vi "Keithley Report2400.vi"(0 "Test operator":string="Operator's name", 1 "Start":string="100", 2 "AppArray":bool[](array[boolean])=[FALSE, FALSE, FALSE, FALSE, FALSE, FALSE, FALSE, FALSE, FALSE, FALSE, FALSE, FALSE, FALSE, FALSE, FALSE, FALSE, FALSE, FALSE, FALSE, FALSE], 3 "Cluster":T1={"A 3"=[["100", "41.7", "38.5"], ["125", "41.7", "35.2"], ["160", "41.5", "37.5"], ["200", "42.3", "42.5"], ["250", "46.9", "46.8"], ["315", "51.9", "52.6"], ["400", "52.3", "46.7"], ["500  ", "46.5", "41.6"], ["630", "42.3", "35.9"], ["800", "41.1", "32.6"]], "A 4"=[["100", "41.7", "38.5"], ["125", "41.7", "35.2"], ["160", "41.5", "37.5"], ["200", "42.3", "42.5"], ["250", "46.9", "46.8"], ["315", "51.9", "52.6"], ["400", "52.3", "46.7"], ["500  ", "46.5", "41.6"], ["630", "42.3", "35.9"], ["800", "41.1", "32.6"]], "A 5"=[["100", "41.7", "38.5"], ["125", "41.7", "35.2"], ["160", "41.5", "37.5"], ["200", "42.3", "42.5"], ["250", "46.9", "46.8"], ["315", "51.9", "52.6"], ["400", "52.3", "46.7"], ["500  ", "46.5", "41.6"], ["630", "42.3", "35.9"], ["800", "41.1", "32.6"]], "A 6"=[["100", "41.7", "38.5"], ["125", "41.7", "35.2"], ["160", "41.5", "37.5"], ["200", "42.3", "42.5"], ["250", "46.9", "46.8"], ["315", "51.9", "52.6"], ["400", "52.3", "46.7"], ["500  ", "46.5", "41.6"], ["630", "42.3", "35.9"], ["800", "41.1", "32.6"]], "A 7"=[["100", "41.7", "38.5"], ["125", "41.7", "35.2"], ["160", "41.5", "37.5"], ["200", "42.3", "42.5"], ["250", "46.9", "46.8"], ["315", "51.9", "52.6"], ["400", "52.3", "46.7"], ["500  ", "46.5", "41.6"], ["630", "42.3", "35.9"], ["800", "41.1", "32.6"]], "A 8"=[["100", "41.7", "38.5"], ["125", "41.7", "35.2"], ["160", "41.5", "37.5"], ["200", "42.3", "42.5"], ["250", "46.9", "46.8"], ["315", "51.9", "52.6"], ["400", "52.3", "46.7"], ["500  ", "46.5", "41.6"], ["630", "42.3", "35.9"], ["800", "41.1", "32.6"]], "A 9"=[["100", "41.7", "38.5"], ["125", "41.7", "35.2"], ["160", "41.5", "37.5"], ["200", "42.3", "42.5"], ["250", "46.9", "46.8"], ["315", "51.9", "52.6"], ["400", "52.3", "46.7"], ["500  ", "46.5", "41.6"], ["630", "42.3", "35.9"], ["800", "41.1", "32.6"]], "A 10"=[["100", "41.7", "38.5"], ["125", "41.7", "35.2"], ["160", "41.5", "37.5"], ["200", "42.3", "42.5"], ["250", "46.9", "46.8"], ["315", "51.9", "52.6"], ["400", "52.3", "46.7"], ["500  ", "46.5", "41.6"], ["630", "42.3", "35.9"], ["800", "41.1", "32.6"]], "A 11"=[["100", "41.7", "38.5"], ["125", "41.7", "35.2"], ["160", "41.5", "37.5"], ["200", "42.3", "42.5"], ["250", "46.9", "46.8"], ["315", "51.9", "52.6"], ["400", "52.3", "46.7"], ["500  ", "46.5", "41.6"], ["630", "42.3", "35.9"], ["800", "41.1", "32.6"]], "A 12"=[["100", "41.7", "38.5"], ["125", "41.7", "35.2"], ["160", "41.5", "37.5"], ["200", "42.3", "42.5"], ["250", "46.9", "46.8"], ["315", "51.9", "52.6"], ["400", "52.3", "46.7"], ["500  ", "46.5", "41.6"], ["630", "42.3", "35.9"], ["800", "41.1", "32.6"]], "A 13"=[["100", "41.7", "38.5"], ["125", "41.7", "35.2"], ["160", "41.5", "37.5"], ["200", "42.3", "42.5"], ["250", "46.9", "46.8"], ["315", "51.9", "52.6"], ["400", "52.3", "46.7"], ["500  ", "46.5", "41.6"], ["630", "42.3", "35.9"], ["800", "41.1", "32.6"]], "A 14"=[["100", "41.7", "38.5"], ["125", "41.7", "35.2"], ["160", "41.5", "37.5"], ["200", "42.3", "42.5"], ["250", "46.9", "46.8"], ["315", "51.9", "52.6"], ["400", "52.3", "46.7"], ["500  ", "46.5", "41.6"], ["630", "42.3", "35.9"], ["800", "41.1", "32.6"]], "A 15"=[["100", "41.7", "38.5"], ["125", "41.7", "35.2"], ["160", "41.5", "37.5"], ["200", "42.3", "42.5"], ["250", "46.9", "46.8"], ["315", "51.9", "52.6"], ["400", "52.3", "46.7"], ["500  ", "46.5", "41.6"], ["630", "42.3", "35.9"], ["800", "41.1", "32.6"]], "A 16"=[["100", "41.7", "38.5"], ["125", "41.7", "35.2"], ["160", "41.5", "37.5"], ["200", "42.3", "42.5"], ["250", "46.9", "46.8"], ["315", "51.9", "52.6"], ["400", "52.3", "46.7"], ["500  ", "46.5", "41.6"], ["630", "42.3", "35.9"], ["800", "41.1", "32.6"]], "A 17"=[["100", "41.7", "38.5"], ["125", "41.7", "35.2"], ["160", "41.5", "37.5"], ["200", "42.3", "42.5"], ["250", "46.9", "46.8"], ["315", "51.9", "52.6"], ["400", "52.3", "46.7"], ["500  ", "46.5", "41.6"], ["630", "42.3", "35.9"], ["800", "41.1", "32.6"]], "A 18"=[["100", "41.7", "38.5"], ["125", "41.7", "35.2"], ["160", "41.5", "37.5"], ["200", "42.3", "42.5"], ["250", "46.9", "46.8"], ["315", "51.9", "52.6"], ["400", "52.3", "46.7"], ["500  ", "46.5", "41.6"], ["630", "42.3", "35.9"], ["800", "41.1", "32.6"]], "A 19"=[["100", "41.7", "38.5"], ["125", "41.7", "35.2"], ["160", "41.5", "37.5"], ["200", "42.3", "42.5"], ["250", "46.9", "46.8"], ["315", "51.9", "52.6"], ["400", "52.3", "46.7"], ["500  ", "46.5", "41.6"], ["630", "42.3", "35.9"], ["800", "41.1", "32.6"]], "A 20"=[["100", "41.7", "38.5"], ["125", "41.7", "35.2"], ["160", "41.5", "37.5"], ["200", "42.3", "42.5"], ["250", "46.9", "46.8"], ["315", "51.9", "52.6"], ["400", "52.3", "46.7"], ["500  ", "46.5", "41.6"], ["630", "42.3", "35.9"], ["800", "41.1", "32.6"]], "A 1"=[["100", "41.7", "38.5"], ["125", "41.7", "35.2"], ["160", "41.5", "37.5"], ["200", "42.3", "42.5"], ["250", "46.9", "46.8"], ["315", "51.9", "52.6"], ["400", "52.3", "46.7"], ["500  ", "46.5", "41.6"], ["630", "42.3", "35.9"], ["800", "41.1", "32.6"]], "A 2"=[["100", "41.7", "38.5"], ["125", "41.7", "35.2"], ["160", "41.5", "37.5"], ["200", "42.3", "42.5"], ["250", "46.9", "46.8"], ["315", "51.9", "52.6"], ["400", "52.3", "46.7"], ["500  ", "46.5", "41.6"], ["630", "42.3", "35.9"], ["800", "41.1", "32.6"]]}, 4 "Stop":string="Operator's name", 5 "Step":string="20", 7 "Compliance":string="70", 8 "Data":string[][](table)=[["100", "41.7", "38.5"], ["125", "41.7", "35.2"], ["160", "41.5", "37.5"], ["200", "42.3", "42.5"], ["250", "46.9", "46.8"], ["315", "51.9", "52.6"], ["400", "52.3", "46.7"], ["500  ", "46.5", "41.6"], ["630", "42.3", "35.9"], ["800", "41.1", "32.6"]], 10 "Comp Unit":string="Operator's name", 11 "DataPoints":string="Operator's name", 12 "Ctl Refnum":refnum<vi>, 13 "Start unit":string="100", 14 "test time":timestamp, 18 "Stop Unit":string="Operator's name", 19 "StepUnit":string="20") -> ()   [LabVIEW 2017]
doc: "This example shows how to generate a report from a template. The template contains a preformatted table and a preformatted graph which are updated with Append Table to Report.vi and Excel Update Graph.vi."
uses:
  <vilib>/addons/_office/_exclsub.llb/font.ctl
  <vilib>/Utility/NIReport.llb/image depth.ctl
  TCH Golbal.vi
  <vilib>/Utility/NIReport.llb/Append Report Text (str wrap).vi
  <vilib>/Utility/NIReport.llb/Append Text Table to Report (wrap).vi
  <vilib>/Utility/NIReport.llb/NI_report.lvclass
  <vilib>/Utility/NIReport.llb/NI_ReportGenerationCore.lvlib
  <vilib>/Utility/NIReport.llb/Excel/NI_Excel.lvclass
  <vilib>/addons/_office/NI_ReportGenerationToolkit.lvlib
panel:
  in  "Express VI?":bool
  # "Overview: This example shows how to generate a report from a template using either the Excel Report Generation VIs or the MS Office Report Express VI.\nRequirements: Report Generation Toolkit, Microsoft Excel\nInstructions:\nRun the VI."
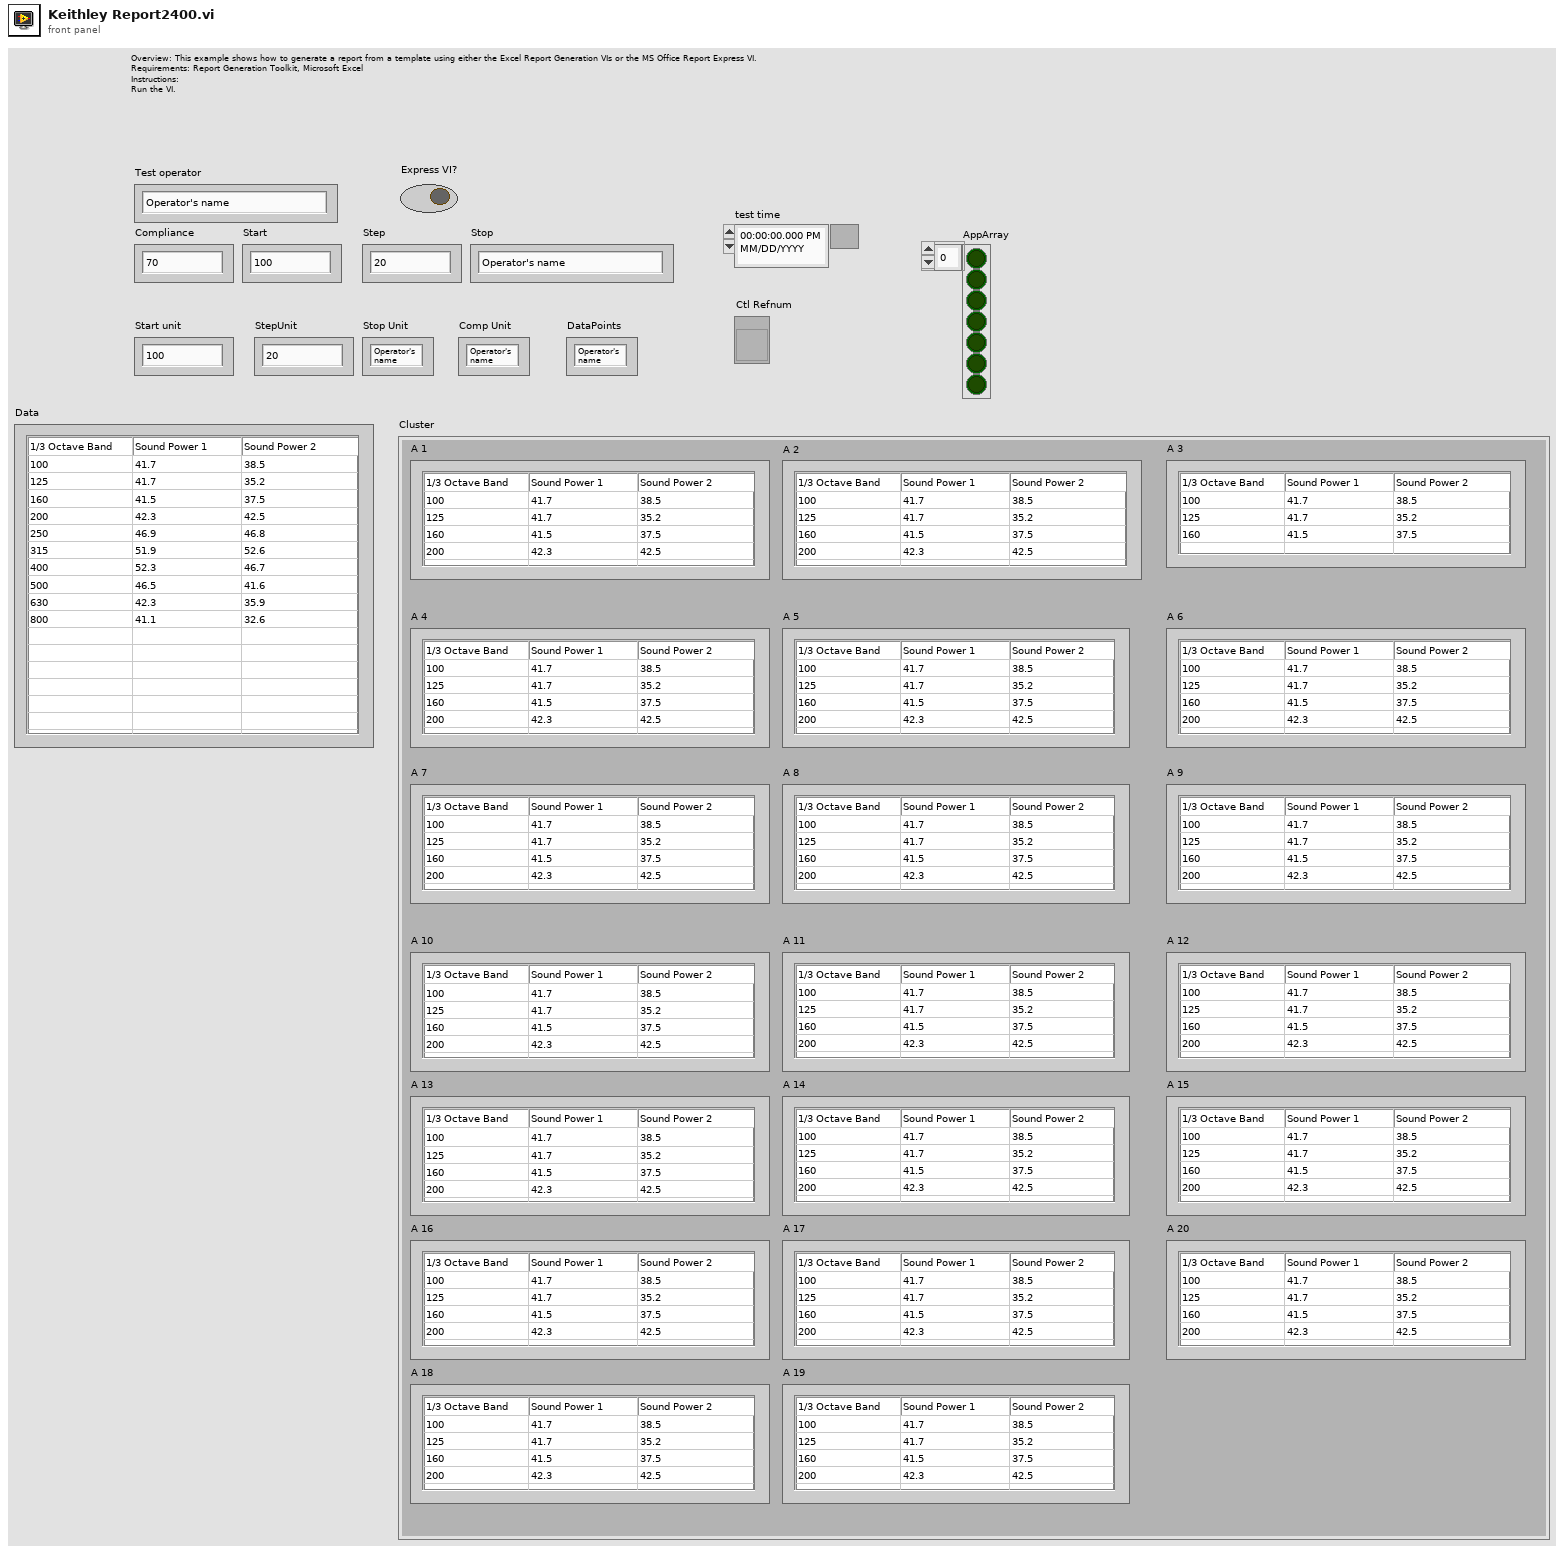
[diagram p1: front panel]
types:
  T1 = cluster{"A 3":string[][], "A 4":string[][], "A 5":string[][], "A 6":string[][], "A 7":string[][], "A 8":string[][], "A 9":string[][], "A 10":string[][], "A 11":string[][], "A 12":string[][], "A 13":string[][], "A 14":string[][], "A 15":string[][], "A 16":string[][], "A 17":string[][], "A 18":string[][], "A 19":string[][], "A 20":string[][], "A 1":string[][], "A 2":string[][]}
  T2 = cluster{"position (Excel)":cluster{"row":i32, "column":i32}, "name (Excel)":string, "bookmark (Word)":string}
  T3 = cluster{"position (excel)":cluster{"row":i32, "column":i32}, "name (excel)":string, "bookmark (word)":string}
  T4 = cluster{"position (Excel)":cluster{"row":i32, "column":i32}, "name (Excel)":string, string}
  T5 = enum16{"Standard Report", "HTML", "Word", "Excel"}
  T6 = enum32{"invalid app kind", "Development System", "Run Time System", "Student Edition", "Embedded LabVIEW", "Evaluation", "Custom"}
  T7 = typedef "NI_ReportGenerationToolkit.lvlib/font.ctl" = cluster{"font name":string, "font size":dbl, "bold":u16, "italic":u16, "underline":u16, "strike through":u16, "font color":u32}
  T8 = cluster{"start (wd) - row (xl) ":i32, "end (wd) - col (xl) ":i32}
  T9 = typedef "NI_ReportGenerationCore.lvlib/image depth.ctl" = u16
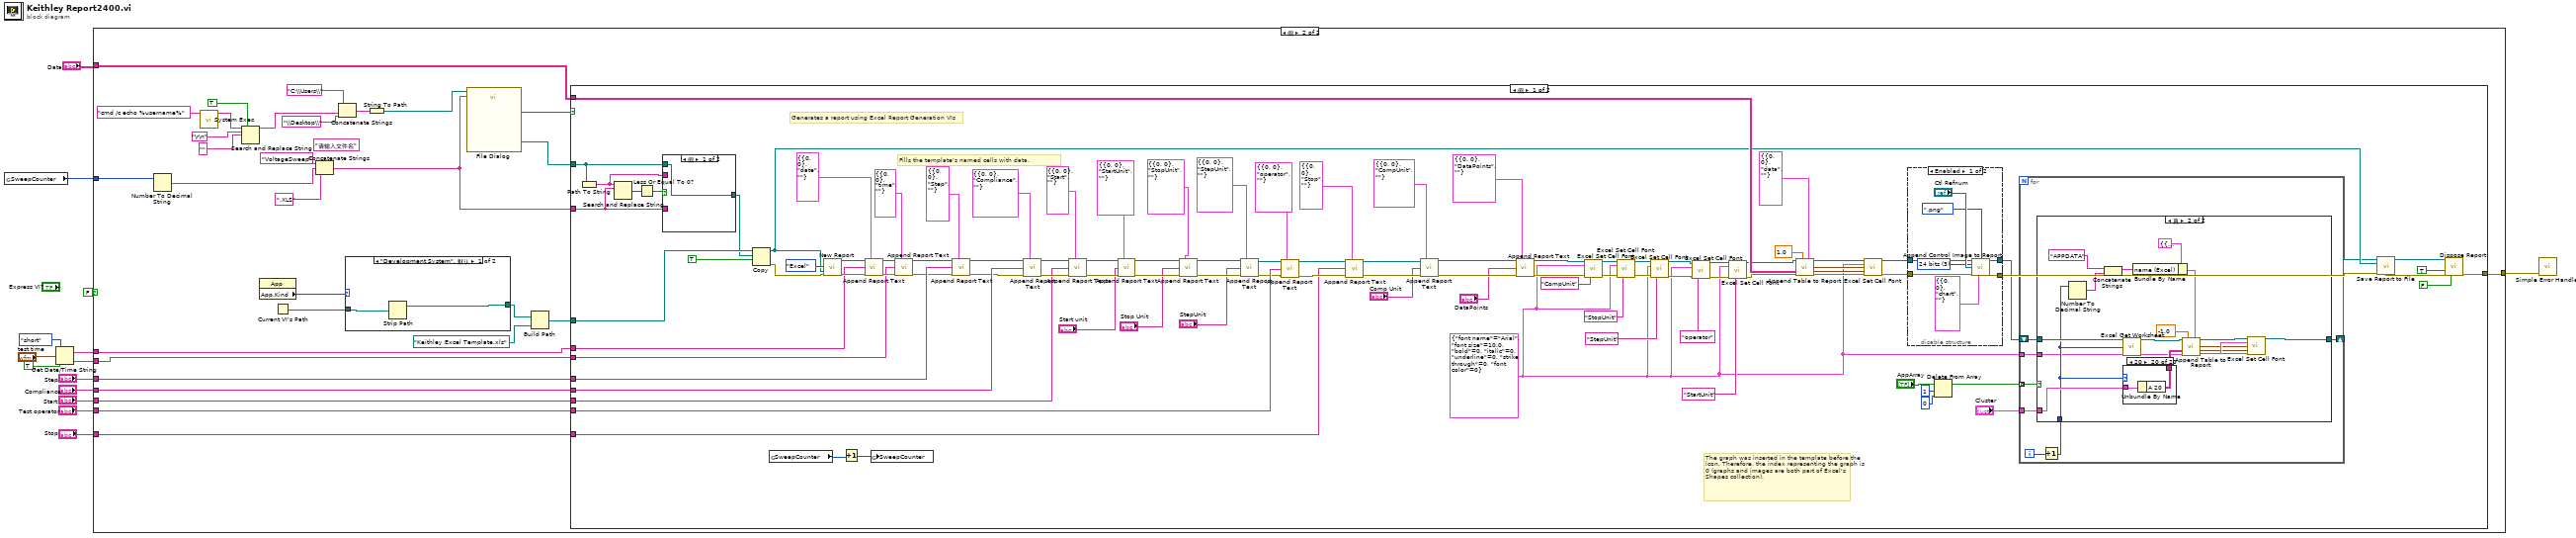
[diagram p0: block diagram]
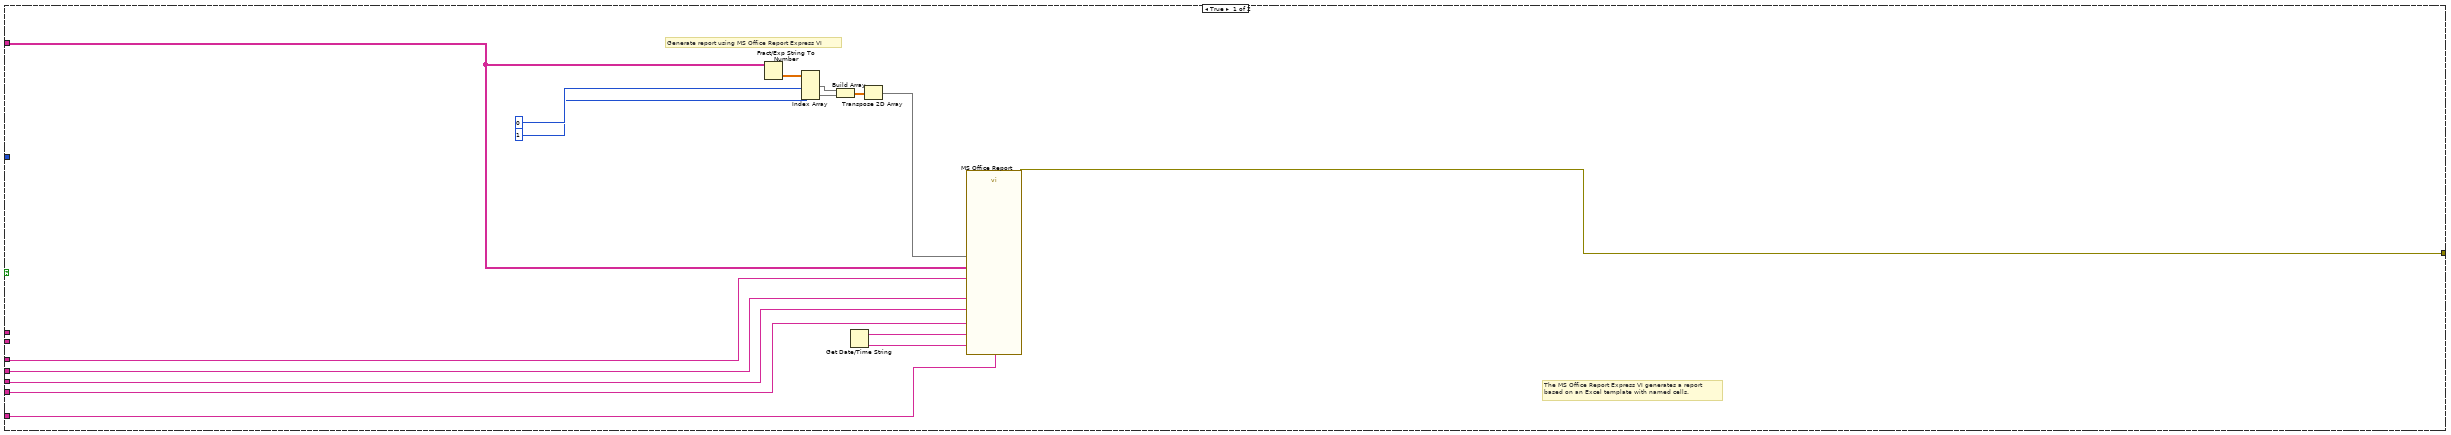
[diagram p2: hidden frame]
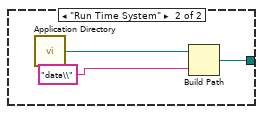
[diagram p3: hidden frame]
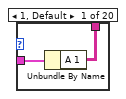
[diagram p6: hidden frame]
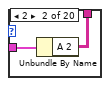
[diagram p7: hidden frame]
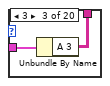
[diagram p8: hidden frame]
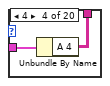
[diagram p9: hidden frame]
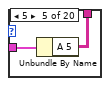
[diagram p10: hidden frame]
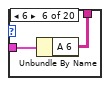
[diagram p11: hidden frame]
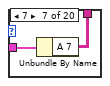
[diagram p12: hidden frame]
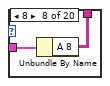
[diagram p13: hidden frame]
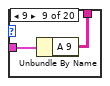
[diagram p14: hidden frame]
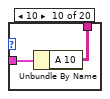
[diagram p15: hidden frame]
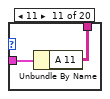
[diagram p16: hidden frame]
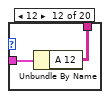
[diagram p17: hidden frame]
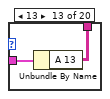
[diagram p18: hidden frame]
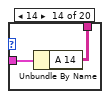
[diagram p19: hidden frame]
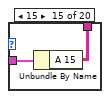
[diagram p20: hidden frame]
diagram:
  n1 = global read "TCH Golbal.vi" "SweepCounter"() -> (w1:i32)
  n2 = Get Date/Time String(date format (0)=enum16{"short", "long", "abbreviated"}."short", seconds (now)="test time", want seconds? (F)=TRUE) -> (date string=w5:string, time string=w4:string)
  n3 = case shown="假" FALSE ("Express VI?") {
    tunnel: "Step" -> [w29 w61]
    tunnel: "Compliance" -> [w23 w60]
    tunnel: "Start" -> [w28 w56]
    tunnel: "Test operator" -> [w27 w55]
    tunnel: [w30 w59] -> w10
    tunnel: "Data" -> [w26 w58]
    tunnel: "Stop" -> [w22 w31]
    tunnel: w5 -> [_ w53]
    tunnel: w4 -> [_ w32]
    tunnel: w1 -> [_ w51]
    frame True {
      # "Generate report using MS Office Report Express VI"
      # "The MS Office Report Express VI generates a report\nbased on an Excel template with named cells."
      n4 = Fract/Exp String To Number(string=w26) -> (number=w21:dbl[][])  [unwired: 3 in, 1 out]
      n5 = Index Array(array=w21, index (col) #1=0 ("disabled index (col)"), index (col) #2=1 ("index (col)")) -> (element #1=w18:dbl[], element #2=w17:dbl[])  [unwired: 2 in]
      n6 = Build Array(w18, w17) -> (w16:dbl[][])
      n7 = Get Date/Time String() -> (date string=w24:string, time string=w25:string)  [unwired: 3 in]
      n8 = Transpose 2D Array(2D array=w16) -> (transposed array=w15:dbl[][])
      n9 = call "MS Office Report"("chart"=w15, "Compliance"=w23, "data"=w26, "date"=w24, "operator"=w27, "Start"=w28, "Step"=w29, "Stop"=w22, "time"=w25) -> ("error out"=w30:errorcluster)  [unwired: 18 in]
    }
    frame False {
      (unwired) "请输入文件名" ("prompt")
      n10 = Number To Decimal String(number=w51) -> (decimal integer string=w50:string)  [unwired: 1 in]
      n11 = call <vilib>:"System Exec.vi"("command line"="cmd /c echo %username%") -> ("standard output"=w42:string)  [unwired: 7 in, 3 out]
      n12 = Search and Replace String(replace all?=TRUE ("replace all? (F)"), input string=w42, search string="\r\n", replace string="" ("replace string (\"\")")) -> (result string=w41:string)  [unwired: 4 in, 3 out]
      n13 = property class="App"() -> ("App.Kind"=w49:T6)  [unwired: 2 in, 2 out]
      n14 = Current VI's Path() -> (path=w34:path)
      n15 = Concatenate Strings("VoltageSweep" ("filename"), w50, ".XLS" ("default name")) -> (w35:string)
      n16 = Concatenate Strings("C:\\Users\\" ("string"), w41, "\\Desktop\\" ("string")) -> (w46:string)
      n17 = case shown="\"Development System\", 默认" w49 {
        tunnel: [w62 w65] -> w33
        tunnel: w34 -> [w63 _]
        frame "Development System", Default {
          n18 = Strip Path(path=w63) -> (stripped path=w62:path)  [unwired: 1 out]
        }
        frame "Run Time System" {
          n19 = call <vilib>:"Application Directory.vi"() -> ("Application Directory"=w64:path)
          n20 = Build Path(base path=w64, name or relative path="data\\") -> (appended path=w65:path)
        }
      }
      n21 = String To Path(string=w46) -> (path=w37:path)
      n22 = call "File Dialog"("start path"=w37, "default name"=w35) -> ("selected path"=w39:path, "cancelled"=w36:bool)  [unwired: 10 in, 2 out]
      n23 = Build Path(base path=w33, name or relative path=path "Keithley Excel Template.xls") -> (appended path=w54:path)
      n24 = case shown="假" w36 {
        tunnel: w61 -> [w167 _]
        tunnel: w60 -> [w166 _]
        tunnel: [w106 _] -> w59
        tunnel: w58 -> [w149 _]
        tunnel: w31 -> [w146 _]
        tunnel: w56 -> [w144 _]
        tunnel: w55 -> [w141 _]
        tunnel: w54 -> [w112 _]
        tunnel: w53 -> [w111 _]
        tunnel: w32 -> [w110 _]
        tunnel: w39 -> [w99 _]
        tunnel: w35 -> [w100 _]
        frame False {
          w67 = T7 {"font name"="Arial", "font size"=10.0, "bold"=0, "italic"=0, "underline"=0, "strike through"=0, "font color"=0} ("font")
          # "Fills the template's named cells with data."
          # "The graph was inserted in the template before the icon. Therefore, the index representing the graph is 0 (graphs and images are both part of Excel's Shapes collection)."
          # "Generates a report using Excel Report Generation VIs"
          n25 = Path To String(path=w99) -> (string=w74:string)
          n26 = Search and Replace String(input string=w74, search string=w100) -> (number of replacements=w97:i32)  [unwired: 6 in, 3 out]
          n27 = Less Or Equal To 0?(x=w97) -> (x <= 0?=w101:bool)
          n28 = case shown="假" w101 {
            tunnel: w99 -> [w242 _]
            tunnel: w100 -> [_ _]
            tunnel: [w242 w243] -> w98
            tunnel: w74 -> [_ w246]
            frame False {
            }
            frame True {
              n29 = Concatenate Strings(w246, ".xls" ("string")) -> (w244:string)
              n30 = String To Path(string=w244) -> (path=w243:path)
            }
          }
          n31 = Copy(9:TRUE ("overwrite (F)"), 10:w98, 11:w112) -> (0:w102:errorcluster, 3:w103:path)  [unwired: 2 in, 1 out]
          n32 = global read "TCH Golbal.vi" "SweepCounter"() -> (w109:i32)
          n33 = call <vilib>:"New Report.vi"("report type"=T5."Excel", "template (empty)"=w103, "error in (no error)"=w102) -> ("report out"=w159:refnum<class "NI_report.lvclass">, "error out"=w164:errorcluster)  [unwired: 11 in]
          n34 = Increment(x=w109) -> (x+1=w108:i32)
          n35 = call-poly <vilib>:"Append Report Text.vi"("report in"=w159, "MS Office parameters"=T2 {"position (Excel)"={"row"=0, "column"=0}, "name (Excel)"="date", "bookmark (Word)"=""}, "text"=w111, "error in (no error)"=w164) -> ("report out"=w158:refnum<class "NI_report.lvclass">, "error out"=w163:errorcluster)  [unwired: 8 in, 2 out]
          n36 = global write "TCH Golbal.vi" "SweepCounter"(w108) -> ()
          n37 = call-poly <vilib>:"Append Report Text.vi"("report in"=w158, "MS Office parameters"=T2 {"position (Excel)"={"row"=0, "column"=0}, "name (Excel)"="time", "bookmark (Word)"=""}, "text"=w110, "error in (no error)"=w163) -> ("report out"=w157:refnum<class "NI_report.lvclass">, "error out"=w162:errorcluster)  [unwired: 8 in, 2 out]
          n38 = call-poly <vilib>:"Append Report Text.vi"("report in"=w157, "MS Office parameters"=T3 {"position (excel)"={"row"=0, "column"=0}, "name (excel)"="Step", "bookmark (word)"=""}, "text"=w167, "error in (no error)"=w162) -> ("report out"=w156:refnum<class "NI_report.lvclass">, "error out"=w161:errorcluster)  [unwired: 8 in, 2 out]
          n39 = call-poly <vilib>:"Append Report Text.vi"("report in"=w156, "MS Office parameters"=T2 {"position (Excel)"={"row"=0, "column"=0}, "name (Excel)"="Compliance", "bookmark (Word)"=""}, "text"=w166, "error in (no error)"=w161) -> ("report out"=w155:refnum<class "NI_report.lvclass">, "error out"=w160:errorcluster)  [unwired: 8 in, 2 out]
          n40 = call-poly <vilib>:"Append Report Text.vi"("report in"=w155, "MS Office parameters"=T2 {"position (Excel)"={"row"=0, "column"=0}, "name (Excel)"="Start", "bookmark (Word)"=""}, "text"=w144, "error in (no error)"=w160) -> ("report out"=w140:refnum<class "NI_report.lvclass">, "error out"=w139:errorcluster)  [unwired: 8 in, 2 out]
          n41 = call-poly <vilib>:"Append Report Text.vi"("report in"=w140, "MS Office parameters"=T3 {"position (excel)"={"row"=0, "column"=0}, "name (excel)"="StartUnit", "bookmark (word)"=""}, "text"="Start unit", "error in (no error)"=w139) -> ("report out"=w138:refnum<class "NI_report.lvclass">, "error out"=w137:errorcluster)  [unwired: 8 in, 2 out]
          n42 = call-poly <vilib>:"Append Report Text.vi"("report in"=w138, "MS Office parameters"=T3 {"position (excel)"={"row"=0, "column"=0}, "name (excel)"="StopUnit", "bookmark (word)"=""}, "text"="Stop Unit", "error in (no error)"=w137) -> ("report out"=w136:refnum<class "NI_report.lvclass">, "error out"=w135:errorcluster)  [unwired: 8 in, 2 out]
          n43 = call-poly <vilib>:"Append Report Text.vi"("report in"=w136, "MS Office parameters"=T3 {"position (excel)"={"row"=0, "column"=0}, "name (excel)"="StepUnit", "bookmark (word)"=""}, "text"="StepUnit", "error in (no error)"=w135) -> ("report out"=w114:refnum<class "NI_report.lvclass">, "error out"=w116:errorcluster)  [unwired: 8 in, 2 out]
          n44 = call-poly <vilib>:"Append Report Text.vi"("report in"=w114, "MS Office parameters"=T2 {"position (Excel)"={"row"=0, "column"=0}, "name (Excel)"="operator", "bookmark (Word)"=""}, "text"=w141, "error in (no error)"=w116) -> ("report out"=w148:refnum<class "NI_report.lvclass">, "error out"=w147:errorcluster)  [unwired: 8 in, 2 out]
          n45 = call-poly <vilib>:"Append Report Text.vi"("report in"=w148, "MS Office parameters"=T2 {"position (Excel)"={"row"=0, "column"=0}, "name (Excel)"="Stop", "bookmark (Word)"=""}, "text"=w146, "error in (no error)"=w147) -> ("report out"=w92:refnum<class "NI_report.lvclass">, "error out"=w91:errorcluster)  [unwired: 8 in, 2 out]
          n46 = call-poly <vilib>:"Append Report Text.vi"("report in"=w92, "MS Office parameters"=T2 {"position (Excel)"={"row"=0, "column"=0}, "name (Excel)"="CompUnit", "bookmark (Word)"=""}, "text"="Comp Unit", "error in (no error)"=w91) -> ("report out"=w94:refnum<class "NI_report.lvclass">, "error out"=w93:errorcluster)  [unwired: 8 in, 2 out]
          n47 = call-poly <vilib>:"Append Report Text.vi"("report in"=w94, "MS Office parameters"=T2 {"position (Excel)"={"row"=0, "column"=0}, "name (Excel)"="DataPoints", "bookmark (Word)"=""}, "text"="DataPoints", "error in (no error)"=w93) -> ("report out"=w88:refnum<class "NI_report.lvclass">, "error out"=w87:errorcluster)  [unwired: 8 in, 2 out]
          n48 = call <vilib>:"Excel Set Cell Font.vi"("report in"=w88, "font"=w67, "error in (no error)"=w87, "name (\"\")"="CompUnit" ("name (\"\")")) -> ("report out"=w86:refnum<class "NI_report.lvclass">, "error out"=w85:errorcluster)  [unwired: 10 in]
          n49 = call <vilib>:"Excel Set Cell Font.vi"("report in"=w86, "font"=w67, "error in (no error)"=w85, "name (\"\")"="StopUnit" ("name (\"\")")) -> ("report out"=w126:refnum<class "NI_report.lvclass">, "error out"=w125:errorcluster)  [unwired: 10 in]
          n50 = call <vilib>:"Excel Set Cell Font.vi"("report in"=w126, "font"=w67, "error in (no error)"=w125, "name (\"\")"="StepUnit" ("name (\"\")")) -> ("report out"=w122:refnum<class "NI_report.lvclass">, "error out"=w123:errorcluster)  [unwired: 10 in]
          n51 = call <vilib>:"Excel Set Cell Font.vi"("report in"=w122, "font"=w67, "error in (no error)"=w123, "name (\"\")"="operator" ("name (\"\")")) -> ("report out"=w121:refnum<class "NI_report.lvclass">, "error out"=w120:errorcluster)  [unwired: 10 in]
          n52 = call <vilib>:"Excel Set Cell Font.vi"("report in"=w121, "font"=w67, "error in (no error)"=w120, "name (\"\")"="StartUnit" ("name (\"\")")) -> ("report out"=w117:refnum<class "NI_report.lvclass">, "error out"=w118:errorcluster)  [unwired: 10 in]
          n53 = call-poly <vilib>:"Append Table to Report.vi"("report in"=w117, "column width (1)"=1.0, "MS Office parameters"=T4 {"position (Excel)"={"row"=0, "column"=0}, "name (Excel)"="data", ""}, "text data"=w149, "error in (no error)"=w118) -> ("report out"=w73:refnum<class "NI_report.lvclass">, "range (wd) - start (xl)"=w69:T8, "end (xl)"=w68:cluster{"row (xl) ":i32, "col (xl) ":i32}, "error out"=w71:errorcluster)  [unwired: 7 in]
          n54 = call <vilib>:"Excel Set Cell Font.vi"("report in"=w73, "font"=w67, "start (-1, -1)"=w69, "end (-1, -1)"=w68, "error in (no error)"=w71) -> ("report out"=w72:refnum<class "NI_report.lvclass">, "error out"=w70:errorcluster)  [unwired: 9 in]
          n55 = disable-structure shown="Enabled" {
            disable-tunnel: [w171 _] -> w105
            disable-tunnel: [w170 w176] -> w82
            disable-tunnel: w72 -> [w169 w176]
            disable-tunnel: w70 -> [w168 _]
            frame Enabled {
              w173 = T9 3 items=["B&W", "4 bits", "8 bits", "24 bits"] ("image depth")
              n56 = call-dynamic "Append Control Image to Report.vi"("report in"=w169, "image file type (.jpg)"=enum16{".jpg", ".png"}.".png", "image depth"=w173, "ctrl reference"="Ctl Refnum", "error in (no error)"=w168, "MS Office parameters"=T2 {"position (Excel)"={"row"=0, "column"=0}, "name (Excel)"="chart", "bookmark (Word)"=""}) -> ("report out"=w170:refnum<class "NI_report.lvclass">, "error out"=w171:errorcluster)  [unwired: 6 in, 2 out]
            }
            frame Disabled {
            }
          }
          n57 = Delete From Array(array="AppArray", length=1, index=0) -> (array with subset deleted=w75:bool[])  [unwired: 1 out]
          n58 = for {
            shift-right: [w182] -> w81
            shift-left: w82 -> [w183]
            tunnel: w75 -> [w181] mode=indexing
            tunnel: "Cluster" -> [w180]
            tunnel: w67 -> [w177]
            i -> [w179]
            n59 = Increment(x=w179) -> (x+1=w178:i32)
            n60 = case shown="真" w181 {
              tunnel: w183 -> [w184 w201]
              tunnel: [w184 w188] -> w182
              tunnel: w180 -> [_ w197]
              tunnel: w178 -> [_ w194]
              tunnel: w177 -> [_ w187]
              frame False {
              }
              frame True {
                n61 = Number To Decimal String(number=w194) -> (decimal integer string=w193:string)  [unwired: 1 in]
                n62 = Concatenate Strings("APPDATA", w193) -> (w191:string)
                n63 = call <vilib>:"Excel Get Worksheet.vi"("report in"=w201, "worksheet index (0)"=w194) -> ("report out"=w200:refnum<class "NI_report.lvclass">)  [unwired: 12 in, 1 out]
                n64 = case shown="20" w194 {
                  tunnel: [w203 w205 w207 w209 w211 w213 w215 w217 w219 w221 w223 w225 w227 w229 w231 w233 w235 w237 w239 w241] -> w199
                  tunnel: w197 -> [w202 w204 w206 w208 w210 w212 w214 w216 w218 w220 w222 w224 w226 w228 w230 w232 w234 w236 w238 w240]
                  frame 1, Default {
                    n65 = Unbundle By Name(w202) -> ("A 1"=w203:string[][])
                  }
                  frame 2 {
                    n66 = Unbundle By Name(w204) -> ("A 2"=w205:string[][])
                  }
                  frame 3 {
                    n67 = Unbundle By Name(w206) -> ("A 3"=w207:string[][])
                  }
                  frame 4 {
                    n68 = Unbundle By Name(w208) -> ("A 4"=w209:string[][])
                  }
                  frame 5 {
                    n69 = Unbundle By Name(w210) -> ("A 5"=w211:string[][])
                  }
                  frame 6 {
                    n70 = Unbundle By Name(w212) -> ("A 6"=w213:string[][])
                  }
                  frame 7 {
                    n71 = Unbundle By Name(w214) -> ("A 7"=w215:string[][])
                  }
                  frame 8 {
                    n72 = Unbundle By Name(w216) -> ("A 8"=w217:string[][])
                  }
                  frame 9 {
                    n73 = Unbundle By Name(w218) -> ("A 9"=w219:string[][])
                  }
                  frame 10 {
                    n74 = Unbundle By Name(w220) -> ("A 10"=w221:string[][])
                  }
                  frame 11 {
                    n75 = Unbundle By Name(w222) -> ("A 11"=w223:string[][])
                  }
                  frame 12 {
                    n76 = Unbundle By Name(w224) -> ("A 12"=w225:string[][])
                  }
                  frame 13 {
                    n77 = Unbundle By Name(w226) -> ("A 13"=w227:string[][])
                  }
                  frame 14 {
                    n78 = Unbundle By Name(w228) -> ("A 14"=w229:string[][])
                  }
                  frame 15 {
                    n79 = Unbundle By Name(w230) -> ("A 15"=w231:string[][])
                  }
                  frame 16 {
                    n80 = Unbundle By Name(w232) -> ("A 16"=w233:string[][])
                  }
                  frame 17 {
                    n81 = Unbundle By Name(w234) -> ("A 17"=w235:string[][])
                  }
                  frame 18 {
                    n82 = Unbundle By Name(w236) -> ("A 18"=w237:string[][])
                  }
                  frame 19 {
                    n83 = Unbundle By Name(w238) -> ("A 19"=w239:string[][])
                  }
                  frame 20 {
                    n84 = Unbundle By Name(w240) -> ("A 20"=w241:string[][])
                  }
                }
                n85 = Bundle By Name(cluster=T2 {"position (Excel)"={"row"=0, "column"=0}, "name (Excel)"="APPDATA1", "bookmark (Word)"=""} ("MS Office parameters"), "name (Excel)"=w191) -> (w195:T2)
                n86 = call-poly <vilib>:"Append Table to Report.vi"("report in"=w200, "column width (1)"=-1.0, "MS Office parameters"=w195, "text data"=w199) -> ("report out"=w189:refnum<class "NI_report.lvclass">, "range (wd) - start (xl)"=w186:T8, "end (xl)"=w185:cluster{"row (xl) ":i32, "col (xl) ":i32}, "error out"=w190:errorcluster)  [unwired: 8 in]
                n87 = call <vilib>:"Excel Set Cell Font.vi"("report in"=w189, "font"=w187, "start (-1, -1)"=w186, "end (-1, -1)"=w185, "error in (no error)"=w190) -> ("report out"=w188:refnum<class "NI_report.lvclass">)  [unwired: 9 in, 1 out]
              }
            }
          }
          n88 = call-dynamic "Save Report to File.vi"("report in"=w81, "report file path"=w103, "error in (no error)"=w105) -> ("report out"=w80:refnum<class "NI_report.lvclass">, "error out"=w104:errorcluster)  [unwired: 11 in]
          n89 = call-dynamic "Dispose Report.vi"("report in"=w80, "save changes? (F)"=TRUE, "error in (no error)"=w104, "close report? (T)"=FALSE ("Close Report? (T)")) -> ("error out"=w106:errorcluster)  [unwired: 11 in]
        }
        frame True {
        }
      }
    }
  }
  n90 = call <vilib>:"Simple Error Handler.vi"("error in (no error)"=w10) -> ()  [unwired: 4 in, 5 out]
